vi "Referenzfahrt starten.vi"(8 "error in (no error)":errorcluster) -> (0 "error out":errorcluster)   [LabVIEW 2014]
uses:
  <vilib>/CANopenLib/CANOPEN.llb/CANopen SDO Create.vi
  <vilib>/CANopenLib/CANOPEN.llb/CANopen SDO Read [U32].vi
  <vilib>/CANopenLib/CANOPEN.llb/CANopen SDO Write [I8].vi
  <vilib>/CANopenLib/CANOPEN.llb/CANopen SDO Write [U16].vi
  <vilib>/CANopenLib/CANOPEN.llb/CANopen SDO Close.vi
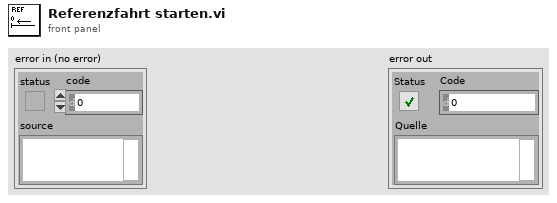
[diagram p1: front panel]
types:
  T1 = enum16{"unbekannt", "Quick stop active", "Fault reaction active", "Fault", "Operation enabled", "Switched on", "Ready to switch on", "Switch on disabled", "Not Ready to switch on"}
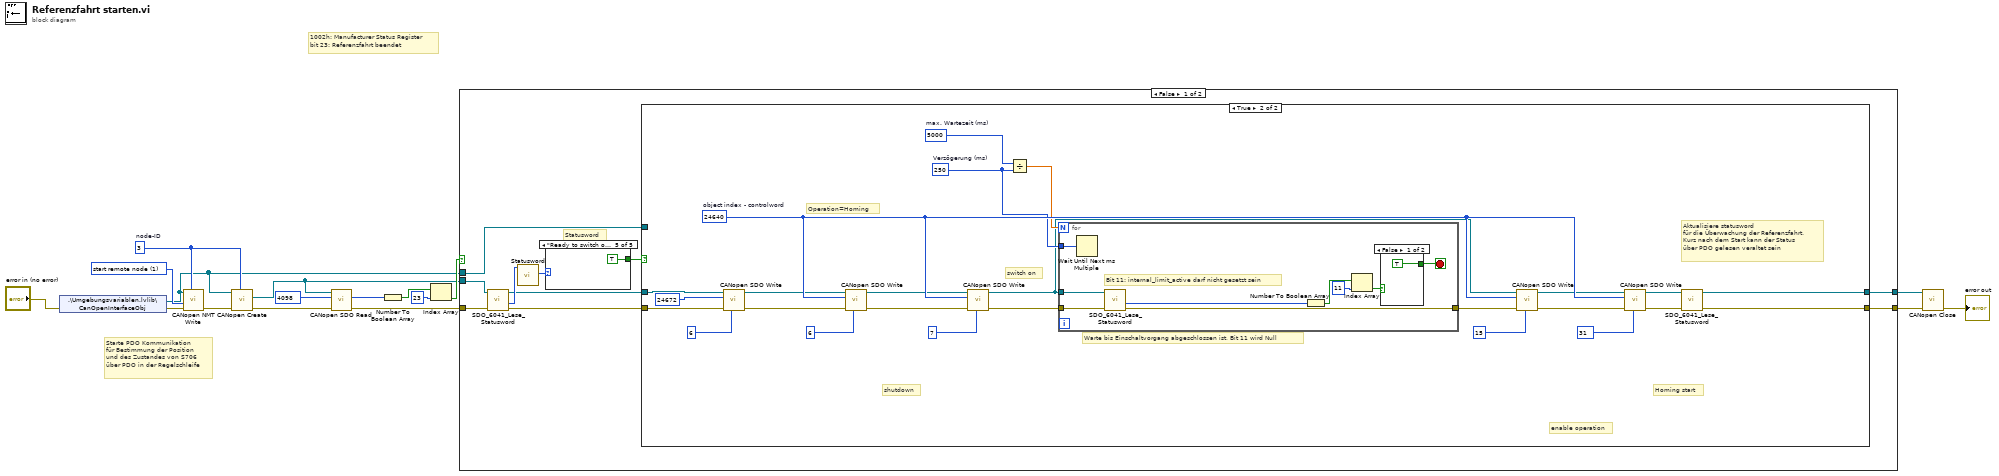
[diagram p0: block diagram]
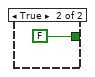
[diagram p3: hidden frame]
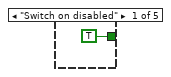
[diagram p4: hidden frame]
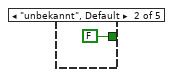
[diagram p5: hidden frame]
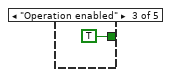
[diagram p6: hidden frame]
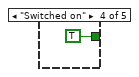
[diagram p7: hidden frame]
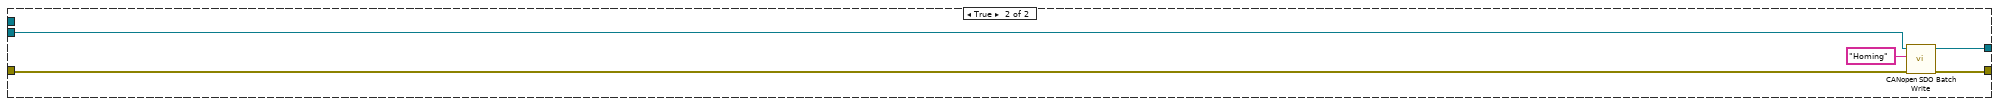
[diagram p8: hidden frame]
diagram:
  w6 = u16 1 items=["start remote node"=1, "stop remote node"=2, "enter pre-operational"=128, "reset node"=129, "reset communication"=130] ("command")
  w5 = u8 3  # node-ID
  # "Starte PDO Kommunikation\nfür Bestimmung der Position\nund des Zustandes von S706\nüber PDO in der Regelschleife"
  # "1002h: Manufacturer Status Register\nbit 23: Referenzfahrt beendet"
  n1 = shared-variable ".\\Umgebungsvariablen.lvlib\\CanOpenInterfaceObj"(error in="error in (no error)") -> (w2:refnum<k20>, error out=w4:errorcluster)
  n2 = call <vilib>:"CANopen NMT Write.vi"("node-ID (0)"=w5, "error in (no error)"=w4, "command"=w6, "interface object in"=w2) -> ("error out"=w3:errorcluster)  [unwired: 6 in, 1 out]
  n3 = call-poly <vilib>:"CANopen Create.vi"("node-ID"=w5, "error in (no error)"=w3, "interface object in"=w2) -> ("error out"=w8:errorcluster, "SDO object out"=w9:refnum<k20>)  [unwired: 6 in, 1 out]
  n4 = call-poly <vilib>:"CANopen SDO Read.vi"("error in (no error)"=w8, "object index"=u16 4098, "SDO object in"=w9) -> ("error out"=w7:errorcluster, "U32 data"=w13:u32)  [unwired: 5 in, 2 out]
  n5 = Number To Boolean Array(number=w13) -> (Boolean array=w12:bool[])
  n6 = Index Array(array=w12, index=23 ("Index")) -> (element=w10:bool)
  n7 = case shown="False" w10 {
    tunnel: w9 -> [w18 w73]
    tunnel: w7 -> [w19 w74]
    tunnel: w2 -> [w25 _]
    tunnel: [w22 w71] -> w16
    tunnel: [w21 w72] -> w15
    frame False {
      # "Statusword"
      n8 = call "SDO_6041_Lese_Statusword.vi"("error in (no error)"=w19, "SDO object in"=w18) -> ("error out"=w23:errorcluster, "U16 data"=w27:u16, "SDO object out"=w24:refnum<k20>)  [unwired: 6 in, 1 out]
      n9 = call "Statusword.vi"("Wert"=w27) -> ("Status"=w26:T1)  [unwired: 10 in]
      n10 = case shown="\"Ready to switch on\"" w26 {
        tunnel: [TRUE FALSE TRUE TRUE TRUE] -> w20
        frame "Switch on disabled" {
        }
        frame "unbekannt", Default {
        }
        frame "Operation enabled" {
        }
        frame "Switched on" {
        }
        frame "Ready to switch on" {
        }
      }
      n11 = case shown="True" w20 {
        tunnel: w25 -> [_ _]
        tunnel: w24 -> [w28 w47]
        tunnel: w23 -> [w29 w30]
        tunnel: [w28 w34] -> w22
        tunnel: [w29 w33] -> w21
        frame False {
        }
        frame True {
          w36 = 250  # Verzögerung (ms)
          w38 = 5000  # max. Wartezeit (ms)
          w52 = u16 24640  # object index - controlword
          # "Aktualisiere statusword \nfür die Überwachung der Referenzfahrt.\nKurz nach dem Start kann der Status \nüber PDO gelesen veraltet sein"
          # "Warte bis Einschaltvorgang abgeschlossen ist, Bit 11 wird Null"
          # "Homing start"
          # "enable operation"
          # "switch on"
          # "shutdown"
          # "Operation=Homing"
          n12 = call-poly <vilib>:"CANopen SDO Write.vi"("I8 data"=i8 6, "error in (no error)"=w30, "object index"=u16 24672, "SDO object in"=w47) -> ("error out"=w42:errorcluster, "SDO object out"=w41:refnum<k20>)  [unwired: 5 in, 1 out]
          n13 = call-poly <vilib>:"CANopen SDO Write.vi"("U16 data"=u16 6, "error in (no error)"=w42, "object index"=w52, "SDO object in"=w41) -> ("error out"=w43:errorcluster, "SDO object out"=w44:refnum<k20>)  [unwired: 5 in, 1 out]
          n14 = call-poly <vilib>:"CANopen SDO Write.vi"("U16 data"=u16 7, "error in (no error)"=w43, "object index"=w52, "SDO object in"=w44) -> ("error out"=w39:errorcluster, "SDO object out"=w31:refnum<k20>)  [unwired: 5 in, 1 out]
          n15 = Divide(x=w38, y=w36) -> (x/y=w37:dbl)
          n16 = for {
            N: w37 -> [_]
            tunnel: [w57] -> w40
            tunnel: w39 -> [w58]
            tunnel: w36 -> [w59]
            tunnel: w31 -> [w56]
            stop <- w60 stop-if-true
            # "Bit 11: internal_limit_active darf nicht gesetzt sein"
            n17 = Wait Until Next ms Multiple(millisecond multiple=w59) -> ()  [unwired: 1 out]
            n18 = call "SDO_6041_Lese_Statusword.vi"("error in (no error)"=w58, "SDO object in"=w56) -> ("error out"=w57:errorcluster, "U16 data"=w55:u16)  [unwired: 6 in, 2 out]
            n19 = Number To Boolean Array(number=w55) -> (Boolean array=w63:bool[])
            n20 = Index Array(array=w63, index=11 ("Index")) -> (element=w61:bool)
            n21 = case shown="False" w61 {
              tunnel: [TRUE FALSE] -> w60
              frame False {
              }
              frame True {
              }
            }
          }
          n22 = call-poly <vilib>:"CANopen SDO Write.vi"("U16 data"=u16 15, "error in (no error)"=w40, "object index"=w52, "SDO object in"=w31) -> ("error out"=w45:errorcluster, "SDO object out"=w46:refnum<k20>)  [unwired: 5 in, 1 out]
          n23 = call-poly <vilib>:"CANopen SDO Write.vi"("U16 data"=u16 31, "error in (no error)"=w45, "object index"=w52, "SDO object in"=w46) -> ("error out"=w32:errorcluster, "SDO object out"=w35:refnum<k20>)  [unwired: 5 in, 1 out]
          n24 = call "SDO_6041_Lese_Statusword.vi"("error in (no error)"=w32, "SDO object in"=w35) -> ("error out"=w33:errorcluster, "SDO object out"=w34:refnum<k20>)  [unwired: 6 in, 2 out]
        }
      }
    }
    frame True {
      n25 = call <vilib>:"CANopen SDO Batch Write.vi"("error in (no error)"=w74, "batch SDO name"="Homing", "SDO object in"=w73) -> ("error out"=w72:errorcluster, "SDO object out"=w71:refnum<k20>)  [unwired: 6 in, 1 out]
    }
  }
  n26 = call-poly <vilib>:"CANopen Close.vi"("error in (no error)"=w15, "SDO object in"=w16) -> ("error out"=→"error out":errorcluster)  [unwired: 9 in]
